vi "Write Execution time.vi"(10 "Execution time (s)":dbl=-1.0, 11 "Properties.Assert in":refnum<class "Properties.Assert.lvclass">) -> (3 "Properties.Assert out":refnum<class "Properties.Assert.lvclass">)   [LabVIEW 2013, in "Caraya.lvlib" / "Properties.Assert.lvclass"]
uses:
  Properties.Assert.lvclass
  Properties.Assert.lvclass/Properties.Assert.ctl
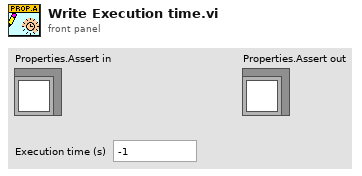
[diagram p1: front panel]
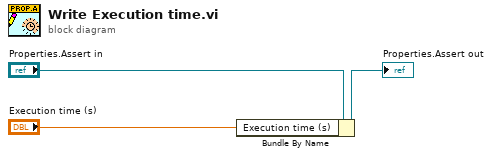
[diagram p0: block diagram]
diagram:
  n1 = Bundle By Name(cluster="Properties.Assert in", "Execution time (s)"="Execution time (s)") -> (→"Properties.Assert out":refnum<class "Properties.Assert.lvclass">)
